vi "Teleop_Turret.vi"(11 "Joystick_IN":T1) -> ()   [LabVIEW 2019]
uses:
  Utility_VIs/Joystick_Controls.ctl
  Turret_Cluster.ctl
  Turret_Globals.vi
panel:
  in  "Spin_Power":dbl
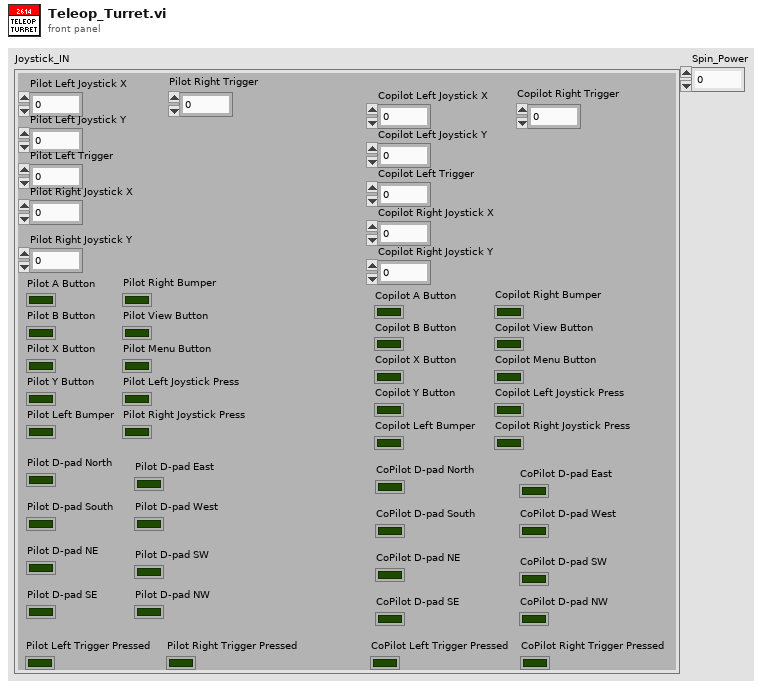
[diagram p1: front panel]
types:
  T1 = typedef "Joystick_Controls.ctl" = cluster{"Pilot Left Joystick X":dbl, "Pilot Left Joystick Y":dbl, "Pilot A Button":bool, "Pilot B Button":bool, "Pilot X Button":bool, "Pilot Y Button":bool, "Pilot Left Bumper":bool, "Pilot Right Bumper":bool, "Pilot View Button":bool, "Pilot Menu Button":bool, "Pilot Left Joystick Press":bool, "Pilot Right Joystick Press":bool, "Pilot Left Trigger":dbl, "Pilot Right Joystick X":dbl, "Pilot Right Joystick Y":dbl, "Pilot Right Trigger":dbl, "Copilot Left Joystick X":dbl, "Copilot Left Joystick Y":dbl, "Copilot A Button":bool, "Copilot B Button":bool, "Copilot X Button":bool, "Copilot Y Button":bool, "Copilot Left Bumper":bool, "Copilot Right Bumper":bool, "Copilot View Button":bool, "Copilot Menu Button":bool, "Copilot Left Joystick Press":bool, "Copilot Right Joystick Press":bool, "Copilot Left Trigger":dbl, "Copilot Right Joystick X":dbl, "Copilot Right Joystick Y":dbl, "Copilot Right Trigger":dbl, "Pilot D-pad North":bool, "Pilot D-pad South":bool, "Pilot D-pad East":bool, "Pilot D-pad West":bool, "Pilot D-pad NE ":bool, "Pilot D-pad SE":bool, "Pilot D-pad SW":bool, "Pilot D-pad NW":bool, "CoPilot D-pad North":bool, "CoPilot D-pad South":bool, "CoPilot D-pad East":bool, "CoPilot D-pad West":bool, "CoPilot D-pad NE":bool, "CoPilot D-pad SE":bool, "CoPilot D-pad SW":bool, "CoPilot D-pad NW":bool, "Pilot Left Trigger Pressed":bool, "Pilot Right Trigger Pressed":bool, "CoPilot Left Trigger Pressed":bool, "CoPilot Right Trigger Pressed":bool}
  T2 = typedef "Turret_Cluster.ctl" = cluster{"Control_State":enum16{"Manual_PercentVoltage", "Manual_SpeedControl", "Auto_Targeting"}, "Spin_Power":dbl, "Flywheel_Power":dbl}
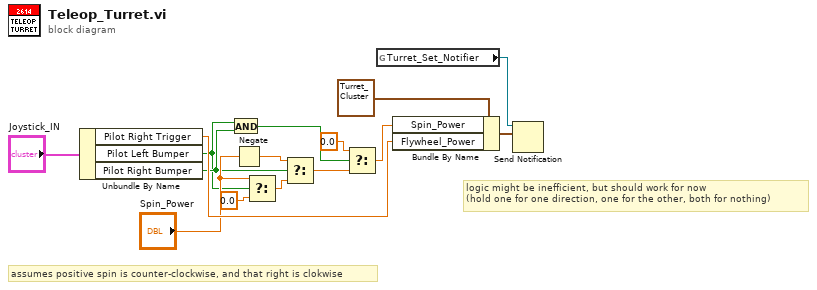
[diagram p0: block diagram]
diagram:
  # "logic might be inefficient, but should work for now\n(hold one for one direction, one for the other, both for nothing)"
  # "assumes positive spin is counter-clockwise, and that right is clokwise"
  n1 = Unbundle By Name("Joystick_IN") -> ("Pilot Right Trigger"=w11:dbl, "Pilot Left Bumper"=w5:bool, "Pilot Right Bumper"=w6:bool)
  n2 = And(x=w5, y=w6) -> (x .and. y?=w4:bool)
  n3 = Negate(x="Spin_Power") -> (-x=w8:dbl)
  n4 = Select(t="Spin_Power", s=w5, f=0.0) -> (s? t:f=w10:dbl)
  n5 = Select(t=w8, s=w6, f=w10) -> (s? t:f=w3:dbl)
  n6 = Select(t=0.0, s=w4, f=w3) -> (s? t:f=w1:dbl)
  n7 = global read "Turret_Globals.vi" "Turret_Set_Notifier"() -> (w14:refnum<notifier>)
  n8 = Bundle By Name(cluster=T2 {"Control_State"=enum."Manual_PercentVoltage", "Spin_Power"=0.0, "Flywheel_Power"=0.0} ("notification"), "Spin_Power"=w1, "Flywheel_Power"=w11) -> (w12:T2)
  n9 = Send Notification(notification=w12, notifier=w14) -> ()  [unwired: 1 in, 2 out]
